vi "CompareStrings.vi"(9 "Expected String":string, 10 "Actual String":string) -> (1 "Message":string, 2 "Equal?":bool)   [LabVIEW 2013, in "UnitTestComparisons.lvlib"]
uses:
  UnitTestComparisons.lvlib
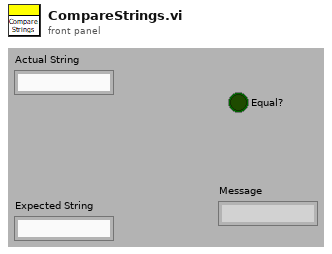
[diagram p1: front panel]
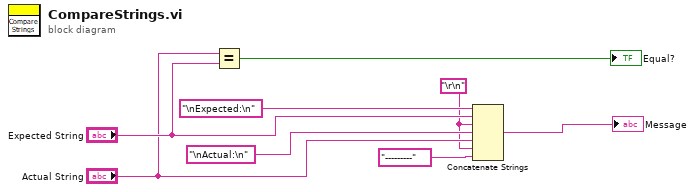
[diagram p0: block diagram]
diagram:
  w1 = "\r\n"
  n1 = Equal?(x="Actual String", y="Expected String") -> (x = y?=→"Equal?":bool)
  n2 = Concatenate Strings("\nExpected:\n" ("string"), "Expected String", w1, "\nActual:\n" ("string"), "Actual String", w1, "---------" ("string")) -> (→"Message":string)
